vi "Write Spectrum Recorder Configuration.vi"(8 "error in (no error)":errorcluster, 10 "Configuration":T1={"Start"=500000.0, "End"=2000000.0, "Duration"=40.0, "Filter time constant"=0.004, "Repeat (-1: forever)"=1, "Update rate"=0.004, "Data storage folder"=path "C:/Data"} {"Update rate" min=0.001 max=10.0 step=0.001 format="%#_6ps"; "Repeat (-1: forever)" format="%.0p"; "Filter time constant" format="%#_6ps"; "Duration" format="%#_6ps"; "End" format="%#_6pHz"; "Start" format="%#_6pHz"}, 11 "Spectrum Recorder in":refnum<class "Spectrum Recorder.lvclass">) -> (0 "error out":errorcluster, 3 "Spectrum Recorder out":refnum<class "Spectrum Recorder.lvclass">)   [LabVIEW 2016, in "Spectrum Recorder.lvclass"]
uses:
  Spectrum Recorder.lvclass
  C:/github/LabActor/Template Module/Template Module.lvclass
  Spectrum Recorder Configuration.ctl
  Template Module/Template Module.lvclass/Template Module.ctl
  Template Module/Write Configuration.vi
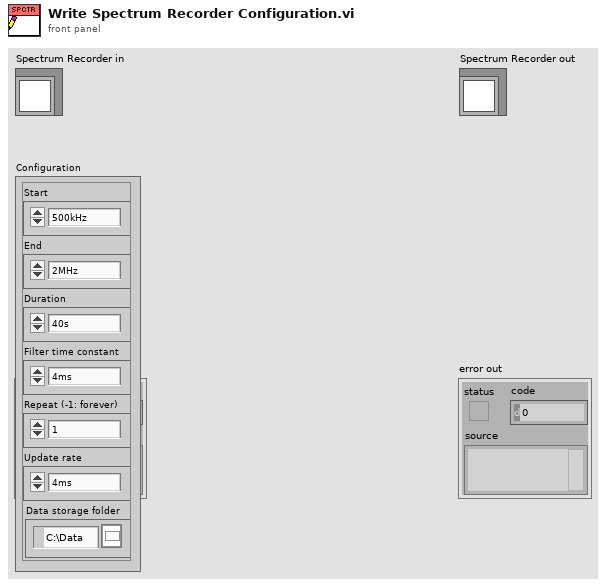
[diagram p1: front panel]
types:
  T1 = typedef "Spectrum Recorder Configuration.ctl" = cluster{"Start":dbl, "End":dbl, "Duration":dbl, "Filter time constant":dbl, "Repeat (-1: forever)":i32, "Update rate":dbl, "Data storage folder":path}
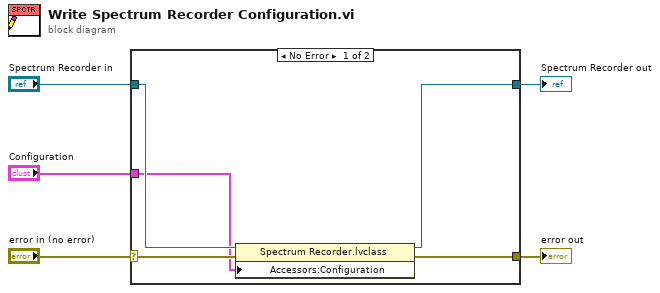
[diagram p0: block diagram]
diagram:
  n1 = case shown="No Error" "error in (no error)" {
    selector: "error in (no error)" -> [w10 w11]
    tunnel: [w9 w11] -> w4
    tunnel: [w7 w12] -> w2
    tunnel: "Spectrum Recorder in" -> [w8 w12]
    tunnel: "Configuration" -> [w6 _]
    frame No Error {
      n2 = property class="Spectrum Recorder.lvclass"(reference=w8, error in=w10, "Accessors:Configuration"=w6) -> (reference out=w7:refnum<class "Spectrum Recorder.lvclass">, error out=w9:errorcluster)
    }
    frame Error {
    }
  }
  "error out" <- w4
  "Spectrum Recorder out" <- w2
